vi "GetUsedTerminalBounds.vi"(4 "SubVI":refnum<vi>) -> (0 "Terminal Bounds[]":T1[](array[typedef]), 1 "VI Name":string, 2 "Terminals[]":refnum<vi>[](array[refnum]))   [LabVIEW 2012]
uses:
  <vilib>/Utility/miscctls.llb/LVRectTypeDef.ctl
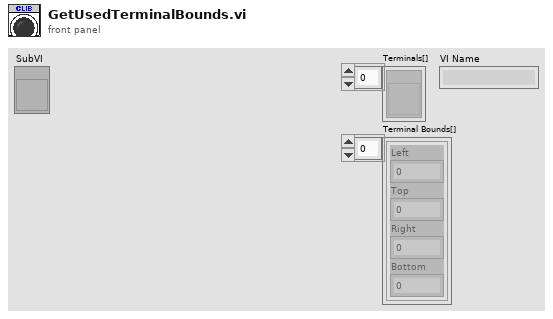
[diagram p1: front panel]
types:
  T1 = typedef "LVRectTypeDef.ctl" = cluster{"Left":i16, "Top":i16, "Right":i16, "Bottom":i16}
  T2 = typedef "NI_XNodeSupport.lvlib/XNodeTerm3.ctl" = cluster{"Name":T3, "Id":T3, "Type":T4, "Bounds":T5, "Input?":T7, "Required?":T7, "Recommended?":T7, "Adaptive?":T7, "Hidden?":T7, "Direction":T8, "Break Wire?":T7}
  T3 = typedef "NI_XNodeSupport.lvlib/XNodeString.ctl" = string
  T4 = typedef "NI_XNodeSupport.lvlib/XNodeVariant.ctl" = variant
  T5 = typedef "NI_XNodeSupport.lvlib/XNodeRect32.ctl" = cluster{"Left":T6, "Top":T6, "Right":T6, "Bottom":T6}
  T6 = typedef "NI_XNodeSupport.lvlib/XNodeInt.ctl" = i32
  T7 = typedef "NI_XNodeSupport.lvlib/XNodeBool.ctl" = bool
  T8 = typedef "NI_XNodeSupport.lvlib/XNodeTermDirection.ctl" = enum32{"Auto", "Up", "Down", "Left", "Right", "Center"}
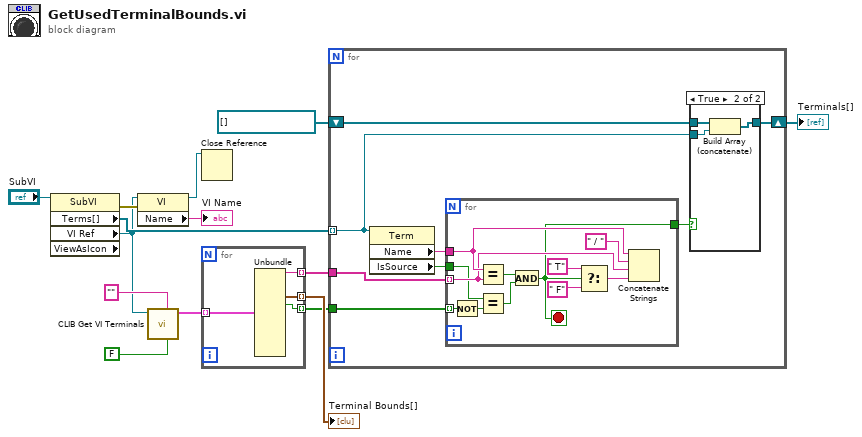
[diagram p0: block diagram]
diagram:
  n1 = property class="SubVI" props=["Terms[]", "VI Ref", "ViewAsIcon"](reference="SubVI") -> (error out=w13:errorcluster, "Terms[]"=w8:refnum<vi>[], "VI Ref"=w3:refnum<vi>)  [unwired: 1 in, 2 out]
  n2 = property class="VI"(reference=w3, error in=w13) -> (reference out=w14:refnum<vi>, "Name"=→"VI Name":string)  [unwired: 1 out]
  n3 = call "CLIB Get VI Terminals.vi"("Clip Edges (T)"=FALSE, "VI-specific ID"="", "reference"=w3) -> ("Terms"=w9:T2[])  [unwired: 7 in, 1 out]
  n4 = Close Reference(reference=w14) -> ()  [unwired: 1 in, 1 out]
  n5 = for {
    tunnel: w9 -> [w18] mode=indexing
    tunnel: [w17] -> w7 mode=indexing
    tunnel: [w16] -> w5 mode=indexing
    tunnel: [w15] -> w2 mode=indexing
    n6 = Unbundle(w18) -> ("Name"=w15:T3, "Bounds"=w17:T5, "Input?"=w16:T7)  [unwired: 8 out]
  }
  "Terminal Bounds[]" <- w7
  n7 = for {
    shift-right: [w24] -> w6
    shift-left: refnum<vi>[] [] -> [w23]
    tunnel: w8 -> [w21] mode=indexing
    tunnel: w5 -> [w19]
    tunnel: w2 -> [w20]
    n8 = property class="Term"(reference=w21) -> ("Name"=w26:string, "IsSource"=w22:bool)  [unwired: 1 in, 2 out]
    n9 = for {
      tunnel: w26 -> [w38]
      tunnel: [w34] -> w25
      tunnel: w22 -> [w35]
      tunnel: w19 -> [w36] mode=indexing
      tunnel: w20 -> [w37] mode=indexing
      stop <- w34 stop-if-true
      n10 = Not(x=w36) -> (.not. x?=w31:T7)
      n11 = Equal?(x=w38, y=w37) -> (x = y?=w33:bool)
      n12 = Equal?(x=w35, y=w31) -> (x = y?=w32:T7)
      n13 = And(x=w33, y=w32) -> (x .and. y?=w34:T7)
      n14 = Select(t=" T" ("Name"), s=w34, f=" F" ("Name")) -> (s? t:f=w42:string)
      n15 = Concatenate Strings(w38, " / " ("string"), w37, w42) -> ()  [unwired: 1 out]
    }
    n16 = case shown="True" w25 {
      tunnel: w21 -> [_ w30]
      tunnel: [w27 w29] -> w24
      tunnel: w23 -> [w27 w28]
      frame False {
      }
      frame True {
        n17 = Build Array (concatenate)(w28, w30) -> (w29:refnum<vi>[])
      }
    }
  }
  "Terminals[]" <- w6
